vi "MAT Save Matrix Header.vi"(4 "Real/Complex (0-Real)":u32, 6 "Rep. Code":u32, 8 "error in (no error)":errorcluster, 9 "Matrix Size":i32[](array[numeric]), 10 "Matrix Name":string, 11 "Ref Num":refnum<file>) -> (0 "error out":errorcluster, 2 "offset":i32, 3 "Dup Ref Num":refnum<file>)   [LabVIEW 2013, in "varilib.lvlib"]
uses:
  varilib.lvlib
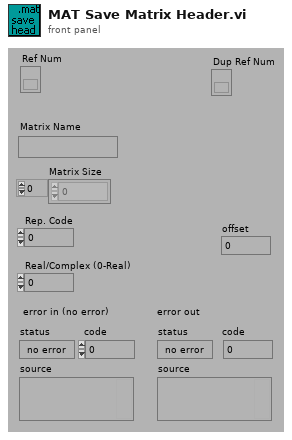
[diagram p1: front panel]
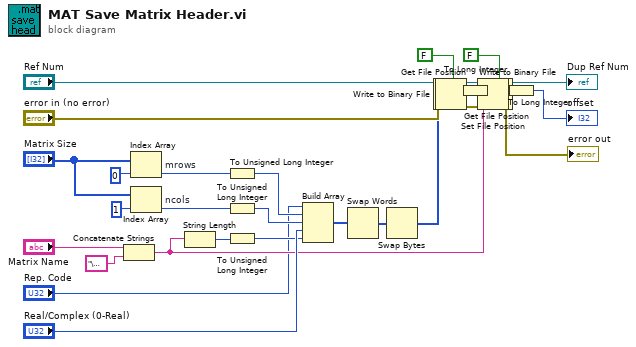
[diagram p0: block diagram]
diagram:
  n1 = Concatenate Strings("Matrix Name", "\u0000") -> (w18:string)
  n2 = Index Array "mrows"(array="Matrix Size", index=0) -> (element=w29:i32)
  n3 = Index Array "ncols"(array="Matrix Size", index=1) -> (element=w30:i32)
  n4 = String Length(string=w18) -> (length=w19:i32)
  n5 = To Unsigned Long Integer(number=w29) -> (unsigned 32bit integer=w28:u32)
  n6 = To Unsigned Long Integer(number=w30) -> (unsigned 32bit integer=w27:u32)
  n7 = To Unsigned Long Integer(number=w19) -> (unsigned 32bit integer=w25:u32)
  n8 = Build Array("Rep. Code", w28, w27, "Real/Complex (0-Real)", w25) -> (w17:u32[])
  n9 = Swap Words(1:w17) -> (0:w16:u32[])
  n10 = Swap Bytes(anything=w16) -> (byte swapped=w15:u32[])
  n11 = Write to Binary File(file (use dialog)="Ref Num", data=w15, error in="error in (no error)", 5:FALSE ("prepend array or string size? (T)")) -> (refnum out=w10:refnum<file>, error out=w9:errorcluster)  [unwired: 2 in, 1 out]
  n12 = Get File Position(4:w9, 7:w10) -> (0:w34:errorcluster, 2:w8:i64, 3:w24:refnum<file>)
  n13 = To Long Integer(number=w8) -> (32bit integer=w22:i32)
  n14 = Set File Position(offset (in bytes) (0)=w22, refnum=w24, error in=w34) -> (refnum out=w6:refnum<file>, error out=w5:errorcluster)  [unwired: 1 in]
  n15 = Write to Binary File(file (use dialog)=w6, data=w18, error in=w5, 5:FALSE ("prepend array or string size? (T)")) -> (refnum out=w4:refnum<file>, error out=w3:errorcluster)  [unwired: 2 in, 1 out]
  n16 = Get File Position(4:w3, 7:w4) -> (0:→"error out":errorcluster, 2:w2:i64, 3:→"Dup Ref Num":refnum<file>)
  n17 = To Long Integer(number=w2) -> (32bit integer=→"offset":i32)
